vi "BXW WXB XWB test.vi"() -> ()   [LabVIEW 2019]
panel:
  out "element 3":string
  out "element 2":string
  out "element":string
  out "white":bool
  out "white 2":bool
  out "toxic 2":bool
  out "toxic":bool
  out "blue 2":bool
  out "blue":bool
  out "Splitted Array":string[](array[string])
  in  "Data":string
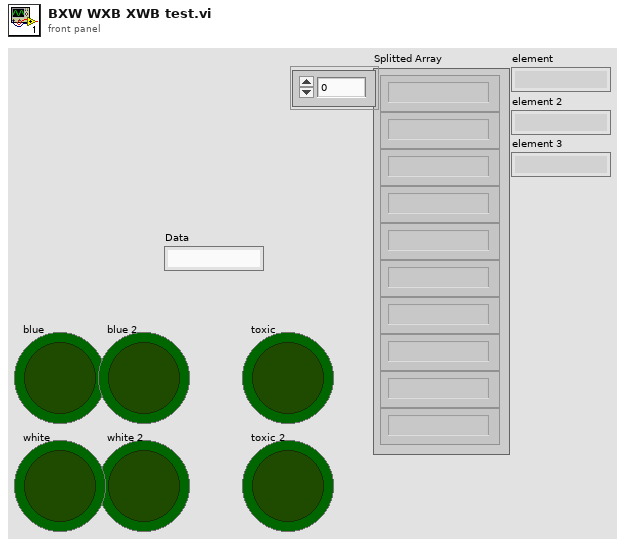
[diagram p1: front panel]
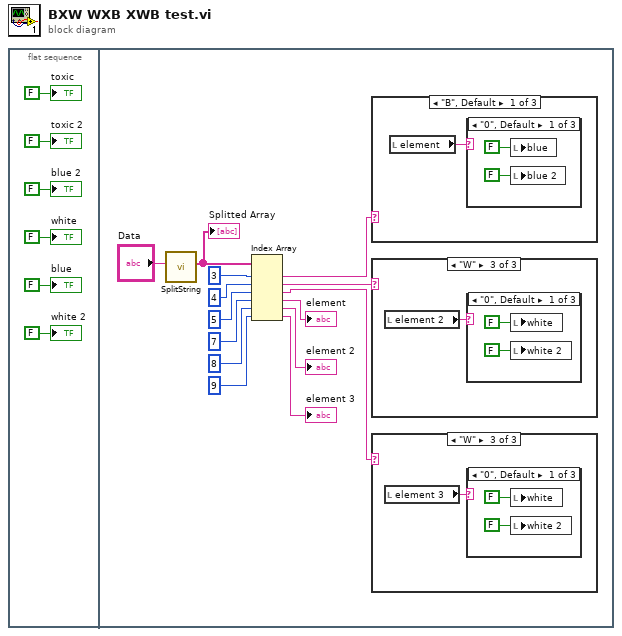
[diagram p0: block diagram]
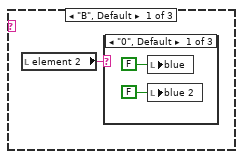
[diagram p2: hidden frame]
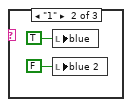
[diagram p3: hidden frame]
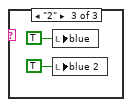
[diagram p4: hidden frame]
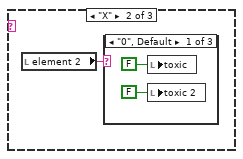
[diagram p5: hidden frame]
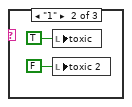
[diagram p6: hidden frame]
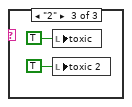
[diagram p7: hidden frame]
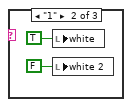
[diagram p8: hidden frame]
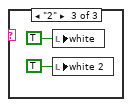
[diagram p9: hidden frame]
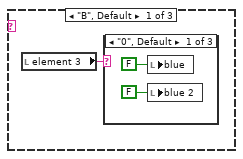
[diagram p10: hidden frame]
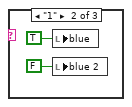
[diagram p11: hidden frame]
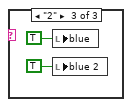
[diagram p12: hidden frame]
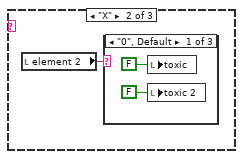
[diagram p13: hidden frame]
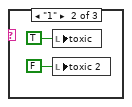
[diagram p14: hidden frame]
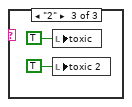
[diagram p15: hidden frame]
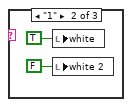
[diagram p16: hidden frame]
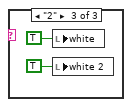
[diagram p17: hidden frame]
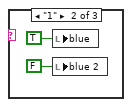
[diagram p18: hidden frame]
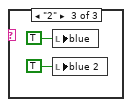
[diagram p19: hidden frame]
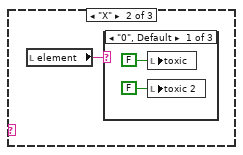
[diagram p20: hidden frame]
diagram:
  n1 = flat-sequence {
    frame #0 {
      "blue" <- FALSE ("blue")
      "blue 2" <- FALSE ("blue 2")
      "toxic" <- FALSE ("toxic")
      "toxic 2" <- FALSE ("toxic 2")
      "white 2" <- FALSE ("white 2")
      "white" <- FALSE ("white")
    }
    frame #1 {
      n2 = call "SplitString.vi"("Data"="Data") -> ("Splitted Array"=w19:string[])  [unwired: 10 in]
      "Splitted Array" <- w19
      n3 = Index Array(array=w19, index #1=3 ("index"), index #2=4 ("index"), index #3=5 ("index"), index #4=7 ("index"), index #5=8 ("index"), index #6=9 ("index")) -> (element #1=w12:string, element #2=w8:string, element #3=w7:string, element #4=→"element":string, element #5=→"element 2":string, element #6=→"element 3":string)
      n4 = case shown="\"B\", Default" w12 {
        frame "B", Default {
          n5 = local read "element"() -> (w63:string)
          n6 = case shown="\"0\", Default" w63 {
            frame "0", Default {
              n7 = local write "blue"(FALSE ("blue")) -> ()
              n8 = local write "blue 2"(FALSE ("blue 2")) -> ()
            }
            frame "1" {
              n9 = local write "blue"(TRUE ("blue")) -> ()
              n10 = local write "blue 2"(FALSE ("blue 2")) -> ()
            }
            frame "2" {
              n11 = local write "blue"(TRUE ("blue")) -> ()
              n12 = local write "blue 2"(TRUE ("blue 2")) -> ()
            }
          }
        }
        frame "X" {
          n13 = local read "element"() -> (w70:string)
          n14 = case shown="\"0\", Default" w70 {
            frame "0", Default {
              n15 = local write "toxic"(FALSE ("blue")) -> ()
              n16 = local write "toxic 2"(FALSE ("blue 2")) -> ()
            }
            frame "1" {
              n17 = local write "toxic"(TRUE ("blue")) -> ()
              n18 = local write "toxic 2"(FALSE ("blue 2")) -> ()
            }
            frame "2" {
              n19 = local write "toxic"(TRUE ("blue")) -> ()
              n20 = local write "toxic 2"(TRUE ("blue 2")) -> ()
            }
          }
        }
        frame "W" {
          n21 = local read "element"() -> (w77:string)
          n22 = case shown="\"0\", Default" w77 {
            frame "0", Default {
              n23 = local write "white"(FALSE ("blue")) -> ()
              n24 = local write "white 2"(FALSE ("blue 2")) -> ()
            }
            frame "1" {
              n25 = local write "white"(TRUE ("blue")) -> ()
              n26 = local write "white 2"(FALSE ("blue 2")) -> ()
            }
            frame "2" {
              n27 = local write "white"(TRUE ("blue")) -> ()
              n28 = local write "white 2"(TRUE ("blue 2")) -> ()
            }
          }
        }
      }
      n29 = case shown="\"W\"" w8 {
        frame "B", Default {
          n30 = local read "element 2"() -> (w21:string)
          n31 = case shown="\"0\", Default" w21 {
            frame "0", Default {
              n32 = local write "blue"(FALSE ("blue")) -> ()
              n33 = local write "blue 2"(FALSE ("blue 2")) -> ()
            }
            frame "1" {
              n34 = local write "blue"(TRUE ("blue")) -> ()
              n35 = local write "blue 2"(FALSE ("blue 2")) -> ()
            }
            frame "2" {
              n36 = local write "blue"(TRUE ("blue")) -> ()
              n37 = local write "blue 2"(TRUE ("blue 2")) -> ()
            }
          }
        }
        frame "X" {
          n38 = local read "element 2"() -> (w28:string)
          n39 = case shown="\"0\", Default" w28 {
            frame "0", Default {
              n40 = local write "toxic"(FALSE ("blue")) -> ()
              n41 = local write "toxic 2"(FALSE ("blue 2")) -> ()
            }
            frame "1" {
              n42 = local write "toxic"(TRUE ("blue")) -> ()
              n43 = local write "toxic 2"(FALSE ("blue 2")) -> ()
            }
            frame "2" {
              n44 = local write "toxic"(TRUE ("blue")) -> ()
              n45 = local write "toxic 2"(TRUE ("blue 2")) -> ()
            }
          }
        }
        frame "W" {
          n46 = local read "element 2"() -> (w35:string)
          n47 = case shown="\"0\", Default" w35 {
            frame "0", Default {
              n48 = local write "white"(FALSE ("blue")) -> ()
              n49 = local write "white 2"(FALSE ("blue 2")) -> ()
            }
            frame "1" {
              n50 = local write "white"(TRUE ("blue")) -> ()
              n51 = local write "white 2"(FALSE ("blue 2")) -> ()
            }
            frame "2" {
              n52 = local write "white"(TRUE ("blue")) -> ()
              n53 = local write "white 2"(TRUE ("blue 2")) -> ()
            }
          }
        }
      }
      n54 = case shown="\"W\"" w7 {
        frame "B", Default {
          n55 = local read "element 3"() -> (w42:string)
          n56 = case shown="\"0\", Default" w42 {
            frame "0", Default {
              n57 = local write "blue"(FALSE ("blue")) -> ()
              n58 = local write "blue 2"(FALSE ("blue 2")) -> ()
            }
            frame "1" {
              n59 = local write "blue"(TRUE ("blue")) -> ()
              n60 = local write "blue 2"(FALSE ("blue 2")) -> ()
            }
            frame "2" {
              n61 = local write "blue"(TRUE ("blue")) -> ()
              n62 = local write "blue 2"(TRUE ("blue 2")) -> ()
            }
          }
        }
        frame "X" {
          n63 = local read "element 2"() -> (w49:string)
          n64 = case shown="\"0\", Default" w49 {
            frame "0", Default {
              n65 = local write "toxic"(FALSE ("blue")) -> ()
              n66 = local write "toxic 2"(FALSE ("blue 2")) -> ()
            }
            frame "1" {
              n67 = local write "toxic"(TRUE ("blue")) -> ()
              n68 = local write "toxic 2"(FALSE ("blue 2")) -> ()
            }
            frame "2" {
              n69 = local write "toxic"(TRUE ("blue")) -> ()
              n70 = local write "toxic 2"(TRUE ("blue 2")) -> ()
            }
          }
        }
        frame "W" {
          n71 = local read "element 3"() -> (w56:string)
          n72 = case shown="\"0\", Default" w56 {
            frame "0", Default {
              n73 = local write "white"(FALSE ("blue")) -> ()
              n74 = local write "white 2"(FALSE ("blue 2")) -> ()
            }
            frame "1" {
              n75 = local write "white"(TRUE ("blue")) -> ()
              n76 = local write "white 2"(FALSE ("blue 2")) -> ()
            }
            frame "2" {
              n77 = local write "white"(TRUE ("blue")) -> ()
              n78 = local write "white 2"(TRUE ("blue 2")) -> ()
            }
          }
        }
      }
    }
  }
